vi "HipEXO_SM_L.vi"(10 "Trigger Ratio":dbl, 11 "Hip Angle":dbl) -> (1 "Boolean":bool, 2 "Boolean 2":bool, 3 "Numeric":dbl)   [LabVIEW 2018]
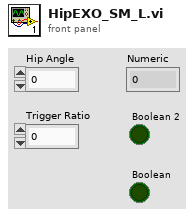
[diagram p1: front panel]
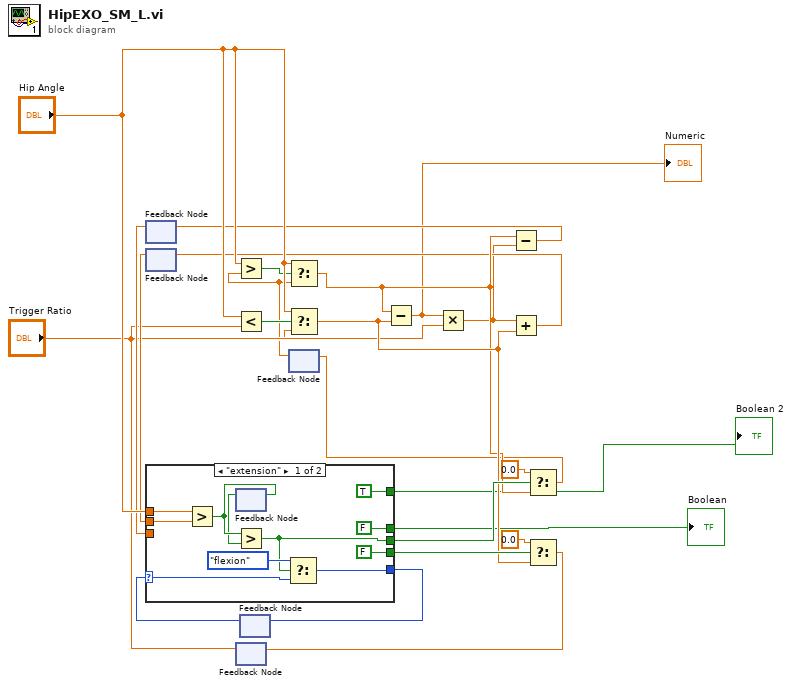
[diagram p0: block diagram]
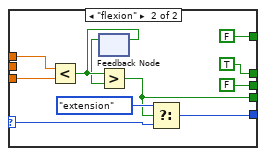
[diagram p2: hidden frame]
diagram:
  n1 = feedback #1() -> (w17:dbl)  [unwired: 1 in]
  n2 = feedback #2() -> (w15:dbl)  [unwired: 1 in]
  n3 = feedback #3() -> (w9:dbl)  [unwired: 1 in]
  n4 = Less?(x="Hip Angle", y=w9) -> (x < y?=w6:bool)
  n5 = feedback #4() -> (w2:enum16{"flexion", "extension"})  [unwired: 1 in]
  n6 = case shown="\"extension\"" w2 {
    selector: w2 -> [w32 w43]
    tunnel: [TRUE FALSE] -> w18
    tunnel: [w33 w44] -> w1
    tunnel: [FALSE TRUE] -> w19
    tunnel: "Hip Angle" -> [w30 w41]
    tunnel: w15 -> [w29 _]
    tunnel: w17 -> [_ w40]
    tunnel: [w25 FALSE ("output")] -> w22
    tunnel: [FALSE ("output") w36] -> w23
    frame "extension" {
      n7 = Greater?(x=w30, y=w29) -> (0:w27:bool)
      n8 = feedback-in #5(w27) -> ()
      n9 = feedback #5() -> (w26:bool)  [unwired: 1 in]
      n10 = Greater?(x=w27, y=w26) -> (0:w25:bool)
      n11 = Select(t=enum16{"flexion", "extension"}."flexion", s=w25, f=w32) -> (s? t:f=w33:enum16{"flexion", "extension"})
    }
    frame "flexion" {
      n12 = Less?(x=w41, y=w40) -> (x < y?=w38:bool)
      n13 = feedback-in #6(w38) -> ()
      n14 = feedback #6() -> (w37:bool)  [unwired: 1 in]
      n15 = Greater?(x=w38, y=w37) -> (0:w36:bool)
      n16 = Select(t=enum16{"flexion", "extension"}."extension", s=w36, f=w43) -> (s? t:f=w44:enum16{"flexion", "extension"})
    }
  }
  "Boolean" <- w19
  "Boolean 2" <- w18
  n17 = feedback-in #4(w1) -> ()
  n18 = Select(t="Hip Angle", s=w6, f=w9) -> (s? t:f=w21:dbl)
  n19 = feedback #7() -> (w5:dbl)  [unwired: 1 in]
  n20 = Greater?(x="Hip Angle", y=w5) -> (0:w4:bool)
  n21 = Select(t="Hip Angle", s=w4, f=w5) -> (s? t:f=w20:dbl)
  n22 = Subtract(x=w20, y=w21) -> (x-y=w13:dbl)
  "Numeric" <- w13
  n23 = Multiply(x=w13, y="Trigger Ratio") -> (x*y=w12:dbl)
  n24 = Subtract(x=w20, y=w12) -> (x-y=w16:dbl)
  n25 = feedback-in #1(w16) -> ()
  n26 = Add(x=w12, y=w21) -> (x+y=w14:dbl)
  n27 = feedback-in #2(w14) -> ()
  n28 = Select(t=0.0, s=w22, f=w20) -> (s? t:f=w10:dbl)
  n29 = feedback-in #7(w10) -> ()
  n30 = Select(t=0.0, s=w23, f=w21) -> (s? t:f=w8:dbl)
  n31 = feedback-in #3(w8) -> ()
